vi "Error_AppendErrorsToSource.vi"(8 "errors in":errorcluster[](array[cluster])) -> (0 "error out":errorcluster)   [LabVIEW 2014, in "hse-misc.lvlib"]
doc: "Takes the first element of <b>errors in</b> and concatenates all other elements' code and source into the source of the first error.\n\n____\nHAMPEL SOFTWARE ENGINEERING v0.7.0 (2018-07-16 18:12)"
uses:
  hse-misc.lvlib
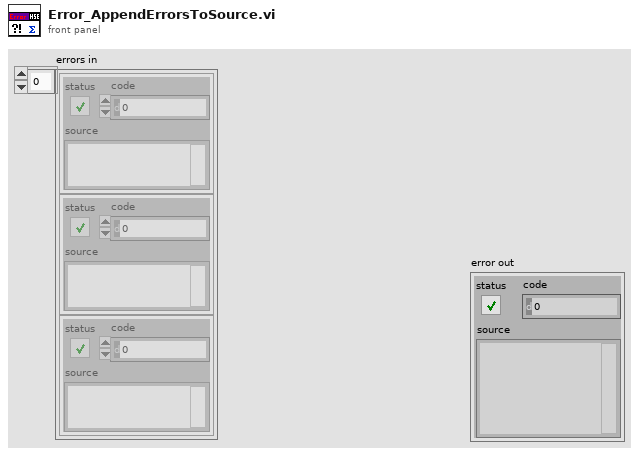
[diagram p1: front panel]
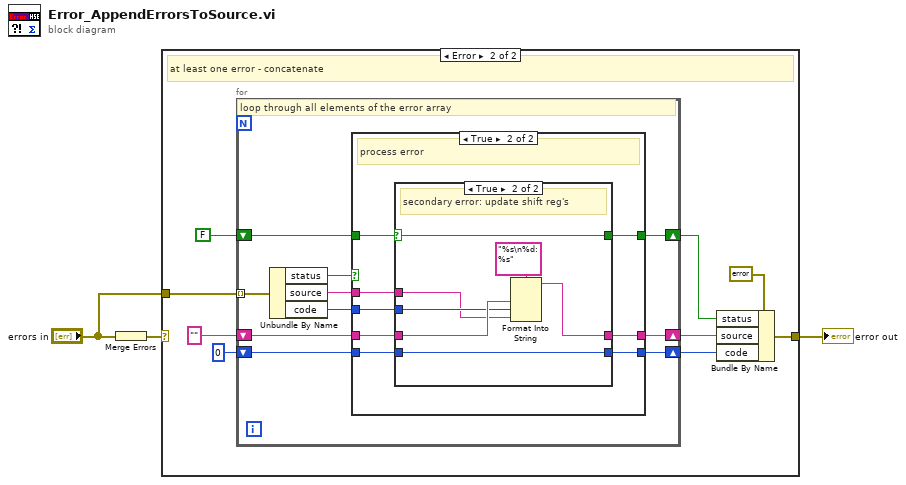
[diagram p0: block diagram]
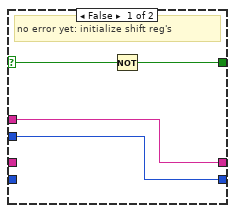
[diagram p4: hidden frame]
diagram:
  n1 = Merge Errors("errors in") -> (w2:errorcluster)
  n2 = case shown="Error" w2 {
    selector: w2 -> [w4 _]
    tunnel: [w4 w13] -> w3
    tunnel: "errors in" -> [_ w11]
    frame No Error {
      # "no error - do nothing"
    }
    frame Error {
      # "at least one error - concatenate"
      n3 = for {
        tunnel: w11 -> [w23] mode=indexing
        shift-right: [w22] -> w5
        shift-left: "" -> [w19]
        shift-right: [w15] -> w10
        shift-left: FALSE -> [w14]
        shift-right: [w16] -> w6
        shift-left: 0 ("code") -> [w17]
        # "loop through all elements of the error array"
        n4 = Unbundle By Name(w23) -> ("status"=w18:bool, "source"=w21:string, "code"=w20:i32)
        n5 = case shown="True" w18 {
          tunnel: [w26 w34] -> w22
          tunnel: w21 -> [_ w33]
          tunnel: w20 -> [_ w32]
          tunnel: w19 -> [w26 w31]
          tunnel: w17 -> [w25 w27]
          tunnel: [w25 w28] -> w16
          tunnel: [w24 w29] -> w15
          tunnel: w14 -> [w24 w30]
          frame False {
            # "no error - keep values"
          }
          frame True {
            # "process error"
            n6 = case shown="True" w30 {
              selector: w30 -> [w38 w41]
              tunnel: [w36 w45] -> w34
              tunnel: w33 -> [w36 w39]
              tunnel: w32 -> [w35 w40]
              tunnel: w31 -> [_ w43]
              tunnel: [w37 w41] -> w29
              tunnel: [w35 w42] -> w28
              tunnel: w27 -> [_ w42]
              frame False {
                # "no error yet: initialize shift reg's"
                n7 = Not(x=w38) -> (.not. x?=w37:bool)
              }
              frame True {
                # "secondary error: update shift reg's"
                n8 = Format Into String(format string="%s\n%d: %s", w43, w40, w39) -> (resulting string=w45:string)  [unwired: 2 in, 1 out]
              }
            }
          }
        }
      }
      n9 = Bundle By Name(cluster=errorcluster {"status"=FALSE, "code"=0, "source"=""} ("error out"), "status"=w10, "source"=w5, "code"=w6) -> (w13:errorcluster)
    }
  }
  "error out" <- w3
